vi "dfd_Get CIC Acc Widths.vi"(5 "Threshold (< 1)":dbl=1.0, 7 "modify?":bool, 11 "multirate filter in":T1={"mMRate_Structure"=enum."CIC", "mMRate_Mode"=0, "mMRate_Factor"=1, "mMRate_FIRParams"={"mMRate_FIR_H"=[], "mMRate_FIR_IsNyquist?"=FALSE, "mMRate_FIR_IsSymmetric?"=FALSE}, "mMRate_CICParams"={"mMRate_CIC_#Stage"=2, "mMRate_CIC_Lag"=1, "mMRate_CIC_Type"=enum."Lowpass"}, "mMRate_Order"=0, "mMRate_Version"="1.0", "mMRate_Comments"="", "mMRate_RationalFactor"={"mMRate_L"=-1, "mMRate_M"=-1}, "mMRate_Fs"=1.0, "mMRate_Quantized?"=FALSE, "mMRate_QFilterGain"=1.0, "mMRate_CoefWl"=16, "mMRate_Scaling"={"mMRate_ScaleByPowerOf2?"=FALSE, "mMRate_ScaleType"=enum."Time Domain 1-Norm"}, "mMRate_InputWl"=0, "mMRate_OutputWl"=0, "mMRate_OutputMode"=enum."Nearest", "mMRate_MultMode"=enum."Truncated", "mMRate_BitPruning"=FALSE, "mMRate_GainWl"=16, "mMRate_OutputFwl"=0, "mMRate_SumIwl"=0, "mMRate_InputIwl "=16, "mMRate_SumWl"=32, "mMRate_CoefIwl"=0} {"mMRate_SumWl" min=1 max=32 step=1; "mMRate_InputIwl" min=1 max=32 step=1; "mMRate_GainWl" min=1 max=32 step=1; "mMRate_OutputWl" min=1 max=32 step=1; "mMRate_InputWl" min=1 max=32 step=1; "mMRate_CoefWl" min=1 max=32 step=1; "mMRate_Mode" items=["Default"=-1, "No Rate Change"=0, "Interpolation"=1, "Decimation"=2, "Interpolated"=3, "Rational"=4]}) -> (0 "sum":dbl, 2 "max Acc width":i16, 3 "Acc width":i32[](array[numeric]))   [LabVIEW 2017, in "NI_DigFilter_FXP.lvlib"]
uses:
  <vilib>/addons/Digital Filter Design/NI_DigFilter_FXP.lvlib
  <vilib>/addons/Digital Filter Design/_Objects.llb/DFD Multirate Filter Obj.ctl
  <vilib>/addons/Digital Filter Design/_Objects.llb/DFD Multirate Mode.ctl
  <vilib>/addons/Digital Filter Design/_Objects.llb/DFD Coef Norm Type.ctl
  <vilib>/addons/Digital Filter Design/_Objects.llb/DFD Round-off Mode.ctl
  <vilib>/addons/Digital Filter Design/_Objects.llb/DFD FXP MRate Multiply Mode.ctl
  <vilib>/addons/Digital Filter Design/Multirate.llb/DFD MRate Filtering (Array).vi
  <vilib>/Analysis/3filter.llb/IIR Filter (DBL).vi
  <vilib>/addons/Digital Filter Design/NI_DigFilterLicensed.lvlib
  <vilib>/Analysis/NI_AALBase.lvlib
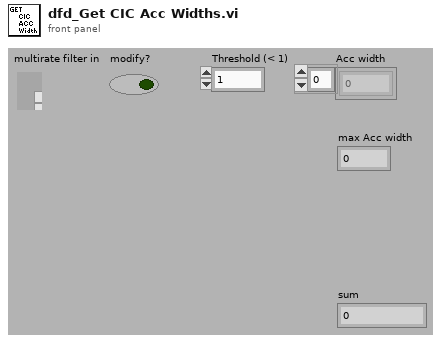
[diagram p1: front panel]
types:
  T1 = typedef "NI_DigFilterLicensed.lvlib/DFD Multirate Filter Obj.ctl" = cluster{"mMRate_Structure":enum16{"CIC", "FIR", "IIR", "Lattice"}, "mMRate_Mode":T2, "mMRate_Factor":i32, "mMRate_FIRParams":cluster{"mMRate_FIR_H":dbl[], "mMRate_FIR_IsNyquist?":bool, "mMRate_FIR_IsSymmetric?":bool}, "mMRate_CICParams":cluster{"mMRate_CIC_#Stage":i32, "mMRate_CIC_Lag":i32, "mMRate_CIC_Type":enum16{"Lowpass", "Highpass"}}, "mMRate_Order":i32, "mMRate_Version":string, "mMRate_Comments":string, "mMRate_RationalFactor":cluster{"mMRate_L":i32, "mMRate_M":i32}, "mMRate_Fs":dbl, "mMRate_Quantized?":bool, "mMRate_QFilterGain":dbl, "mMRate_CoefWl":i16, "mMRate_Scaling":cluster{"mMRate_ScaleByPowerOf2?":bool, "mMRate_ScaleType":T3}, "mMRate_InputWl":i16, "mMRate_OutputWl":i16, "mMRate_OutputMode":T4, "mMRate_MultMode":T5, "mMRate_BitPruning":bool, "mMRate_GainWl":i16, "mMRate_OutputFwl":i16, "mMRate_SumIwl":i16, "mMRate_InputIwl ":i16, "mMRate_SumWl":i16, "mMRate_CoefIwl":i16}
  T2 = typedef "NI_DigFilterLicensed.lvlib/DFD Multirate Mode.ctl" = i16
  T3 = typedef "NI_DigFilterLicensed.lvlib/DFD Coef Norm Type.ctl" = enum16{"No Norm", "Time Domain 1-Norm", "Time Domain 2-Norm", "Time Domain Inf-Norm"}
  T4 = typedef "NI_DigFilterLicensed.lvlib/DFD Round-off Mode.ctl" = enum16{"Nearest", "Truncation"}
  T5 = typedef "NI_DigFilterLicensed.lvlib/DFD FXP MRate Multiply Mode.ctl" = enum16{"Truncated", "Full"}
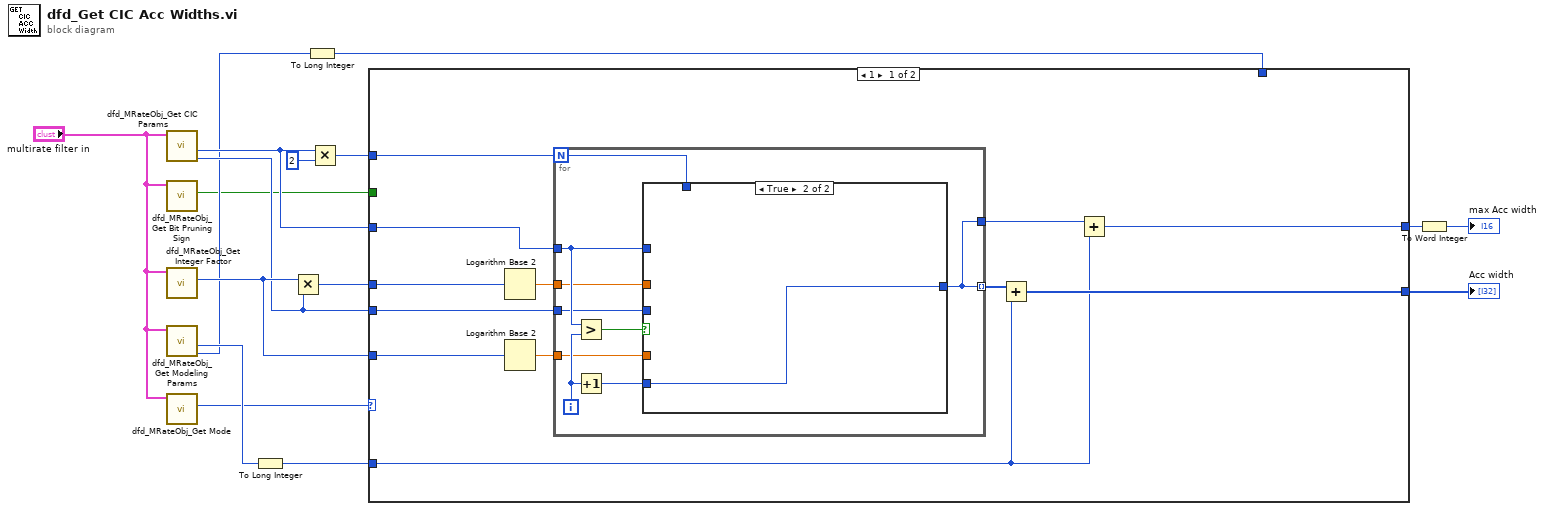
[diagram p0: block diagram]
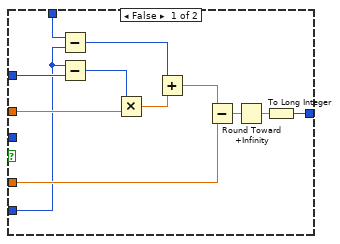
[diagram p2: hidden frame]
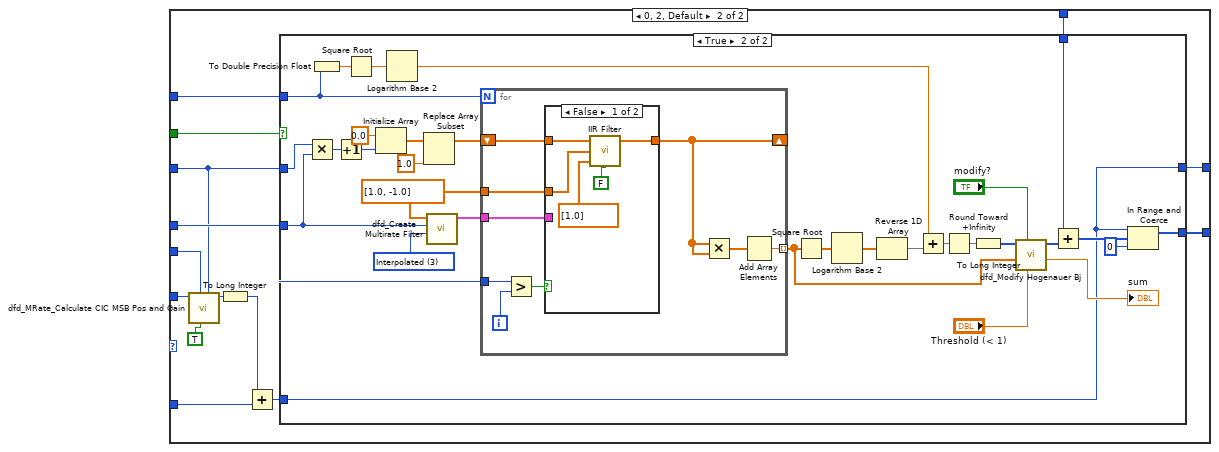
[diagram p3: hidden frame]
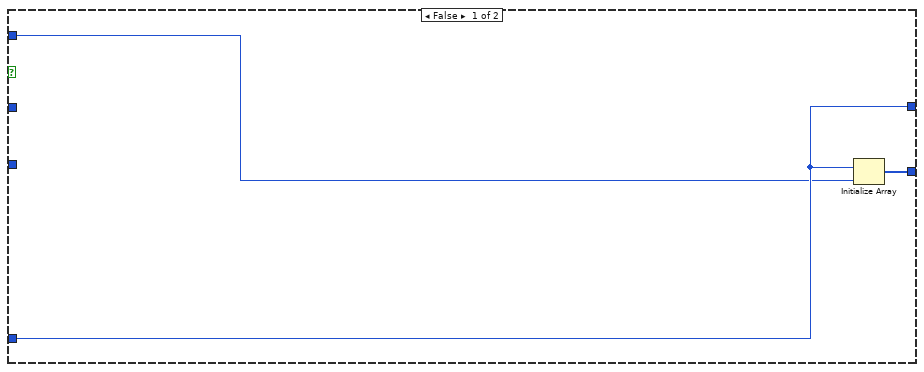
[diagram p4: hidden frame]
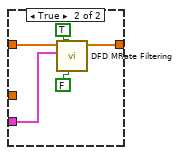
[diagram p5: hidden frame]
diagram:
  n1 = call <vilib>:"dfd_MRateObj_Get CIC Params.vi"("multirate filter in"="multirate filter in") -> ("lag"=w9:i32, "# stages"=w11:i32)  [unwired: 9 out]
  n2 = call <vilib>:"dfd_MRateObj_Get Bit Pruning Sign.vi"("multirate filter in"="multirate filter in") -> ("bit pruning?"=w3:bool)  [unwired: 10 out]
  n3 = call <vilib>:"dfd_MRateObj_Get Integer Factor.vi"("multirate filter in"="multirate filter in") -> ("factor"=w10:i32)  [unwired: 10 out]
  n4 = call <vilib>:"dfd_MRateObj_Get Modeling Params.vi"("multirate filter in"="multirate filter in") -> ("output wl"=w7:i16, "input wl"=w8:i16)  [unwired: 9 out]
  n5 = call <vilib>:"dfd_MRateObj_Get Mode.vi"("multirate filter in"="multirate filter in") -> ("mode"=w6:T2)  [unwired: 10 out]
  n6 = To Long Integer(number=w8) -> (32bit integer=w4:i32)
  n7 = Multiply(x=w10, y=w9) -> (x*y=w14:i32)
  n8 = To Long Integer(number=w7) -> (32bit integer=w5:i32)
  n9 = Multiply(x=w11, y=2) -> (x*y=w15:i32)
  n10 = case shown="1" w6 {
    tunnel: w15 -> [w28 w55]
    tunnel: w14 -> [w27 w59]
    tunnel: w10 -> [w26 w64]
    tunnel: [w22 w54] -> w13
    tunnel: w4 -> [w18 w61]
    tunnel: w9 -> [w21 w63]
    tunnel: w11 -> [w20 w58]
    tunnel: w5 -> [_ w57]
    tunnel: [w17 w51] -> w12
    tunnel: w3 -> [_ w52]
    frame 1 {
      n11 = Logarithm Base 2(1:w27) -> (0:w24:dbl)
      n12 = Logarithm Base 2(1:w26) -> (0:w25:dbl)
      n13 = for {
        N: w28 -> [w30]
        tunnel: w20 -> [w34]
        tunnel: w21 -> [w33]
        tunnel: [w29] -> w23 mode=indexing
        tunnel: w25 -> [w32]
        tunnel: w24 -> [w31]
        tunnel: [w29] -> w19
        i -> [w36]
        n14 = Greater?(x=w34, y=w36) -> (0:w37:bool)
        n15 = Increment(x=w36) -> (x+1=w35:i32)
        n16 = case shown="True" w37 {
          tunnel: w35 -> [w38 w50]
          tunnel: w34 -> [w39 _]
          tunnel: w33 -> [_ _]
          tunnel: [w40 w50] -> w29
          tunnel: w32 -> [w43 _]
          tunnel: w31 -> [w48 _]
          tunnel: w30 -> [w49 _]
          frame False {
            n17 = Subtract(x=w49, y=w38) -> (x-y=w46:i32)
            n18 = Subtract(x=w38, y=w39) -> (x-y=w47:i32)
            n19 = Multiply(x=w47, y=w48) -> (x*y=w45:dbl)
            n20 = Add(x=w46, y=w45) -> (x+y=w44:dbl)
            n21 = Subtract(x=w44, y=w43) -> (x-y=w41:dbl)
            n22 = Round Toward +Infinity(x=w41) -> (ceil(x): smallest int >= x=w42:dbl)
            n23 = To Long Integer(number=w42) -> (32bit integer=w40:i32)
          }
          frame True {
          }
        }
      }
      n24 = Add(x=w23, y=w18) -> (x+y=w22:i32[])
      n25 = Add(x=w19, y=w18) -> (x+y=w17:i32)
    }
    frame 0, 2, Default {
      n26 = call <vilib>:"dfd_MRate_Calculate CIC MSB Pos and Gain.vi"("#stage"=w58, "Decimation? (T)"=TRUE, "lag"=w63, "factor"=w64) -> ("bit growth"=w60:i16)  [unwired: 7 out]
      n27 = To Long Integer(number=w60) -> (32bit integer=w56:i32)
      n28 = Add(x=w56, y=w61) -> (x+y=w53:i32)
      n29 = case shown="True" w52 {
        tunnel: w59 -> [_ w93]
        tunnel: w58 -> [_ w89]
        tunnel: w57 -> [_ w84]
        tunnel: w55 -> [w66 w77]
        tunnel: [w65 w69] -> w54
        tunnel: w53 -> [w67 w68]
        tunnel: [w67 w68] -> w51
        frame False {
          n30 = Initialize Array(w67, w66) -> (w65:i32[])
        }
        frame True {
          w92 = T2 3 items=["Default"=-1, "No Rate Change"=0, "Interpolation"=1, "Decimation"=2, "Interpolated"=3, "Rational"=4] ("mode")
          w90 = dbl[] [1.0, -1.0]
          n31 = Multiply(x=w89, y=w93) -> (x*y=w88:i32)
          n32 = To Double Precision Float(number=w77) -> (double precision float=w81:dbl)
          n33 = Increment(x=w88) -> (x+1=w98:i32)
          n34 = Square Root(x=w81) -> (sqrt(x)=w80:dbl)
          n35 = Initialize Array(0.0 ("element"), w98) -> (w96:dbl[])
          n36 = Logarithm Base 2(1:w80) -> (0:w87:dbl)
          n37 = Replace Array Subset(array=w96, new element=1.0 ("new element/subarray")) -> (w94:dbl[])  [unwired: 1 in]
          n38 = call <vilib>:"dfd_Create Multirate Filter.vi"("mode"=w92, "factor"=w93, "h (n)"=w90) -> ("multirate filter out"=w91:T1)  [unwired: 2 in, 6 out]
          n39 = for {
            N: w77 -> [_]
            shift-right: [w101] -> _
            shift-left: w94 -> [w104]
            tunnel: w91 -> [w103]
            tunnel: w90 -> [w102]
            tunnel: w89 -> [w107]
            tunnel: [w99] -> w75 mode=indexing
            i -> [w106]
            n40 = Greater?(x=w107, y=w106) -> (0:w105:bool)
            n41 = case shown="False" w105 {
              tunnel: w104 -> [w112 w117]
              tunnel: w103 -> [_ w116]
              tunnel: [w110 w113] -> w101
              tunnel: w102 -> [w109 _]
              frame False {
                n42 = call-poly <vilib>:"IIR Filter.vi"("init/cont (init:F)"=FALSE, "Forward Coefficients"=dbl[] [1.0], "Reverse Coefficients"=w109, "X"=w112) -> ("Filtered X"=w110:dbl[])  [unwired: 1 out]
              }
              frame True {
                n43 = call-poly <vilib>:"DFD MRate Filtering.vi"("zero phase? (T)"=FALSE, "init? (F)"=TRUE, "multirate filter"=w116, "signal in"=w117) -> ("signal out"=w113:dbl[])  [unwired: 1 in, 6 out]
              }
            }
            n44 = Multiply(x=w101, y=w101) -> (x*y=w100:dbl[])
            n45 = Add Array Elements(numeric array=w100) -> (sum=w99:dbl)
          }
          n46 = Square Root(x=w75) -> (sqrt(x)=w79:dbl[])
          n47 = Logarithm Base 2(1:w79) -> (0:w78:dbl[])
          n48 = Reverse 1D Array(array=w78) -> (reversed array=w82:dbl[])
          n49 = Add(x=w87, y=w82) -> (x+y=w86:dbl[])
          n50 = Round Toward +Infinity(x=w86) -> (ceil(x): smallest int >= x=w85:dbl[])
          n51 = To Long Integer(number=w85) -> (32bit integer=w72:i32[])
          n52 = call <vilib>:"dfd_Modify Hogenauer Bj.vi"("Threshold (< 1)"="Threshold (< 1)", "modify?"="modify?", "Fj"=w75, "Hogenauer Bj"=w72) -> ("sum"=→"sum":dbl, "output Bj"=w71:i32[])  [unwired: 6 out]
          n53 = Add(x=w84, y=w71) -> (x+y=w70:i32[])
          n54 = In Range and Coerce(upper limit=w68, x=w70, lower limit=0) -> (coerced(x)=w69:i32[])  [unwired: 1 out]
        }
      }
    }
  }
  "Acc width" <- w13
  n55 = To Word Integer(number=w12) -> (16bit integer=→"max Acc width":i16)
